vi "HAL camera initialize - SubVI.vi"() -> (0 "error out":errorcluster)   [LabVIEW 2014]
uses:
  ATMCD32D.DLL
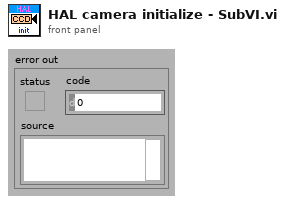
[diagram p1: front panel]
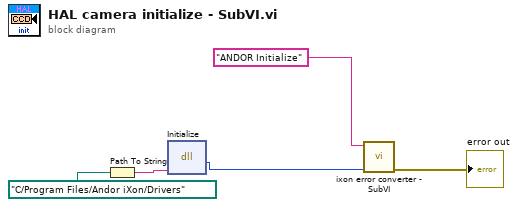
[diagram p0: block diagram]
diagram:
  n1 = Path To String(path=path "C:/Program Files/Andor iXon/Drivers" ("ixon driver directory")) -> (string=w5:string)
  n2 = dll-call lib="ATMCD32D.DLL" fn="Initialize" label="Call Library Function Initialize"(w5) -> (w1:u32)  [unwired: 3 in, 3 out]
  n3 = call "ixon error converter - SubVI.vi"("Andor error code"=w1, "source"="ANDOR Initialize") -> ("error out"=→"error out":errorcluster)  [unwired: 5 in]
